vi "AddModifiers.vi"(8 "Rotation (0=none)":u8, 9 "ColorToReplace (7=white)":fxp<+,3,3>=7.0, 10 "ReplaceColor (1=red)":fxp<+,3,3>=1.0, 11 "String in":string) -> (3 "String out":string)   [LabVIEW 2019, in "RT_Game.lvlib" / "Game.lvclass"]
uses:
  Game/Game.lvclass
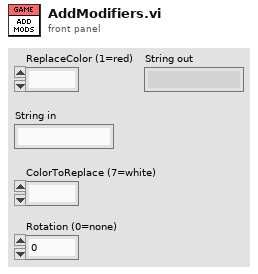
[diagram p1: front panel]
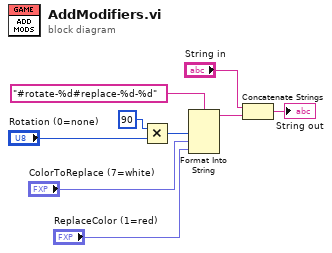
[diagram p0: block diagram]
diagram:
  n1 = Multiply(x=u16 90, y="Rotation (0=none)") -> (x*y=w2:u16)
  n2 = Format Into String(format string="#rotate-%d#replace-%d-%d", w2, "ColorToReplace (7=white)", "ReplaceColor (1=red)") -> (resulting string=w3:string)  [unwired: 2 in, 1 out]
  n3 = Concatenate Strings("String in", w3) -> (→"String out":string)
